vi "MPP.read.vi"(8 "error in (no error)":errorcluster, 11 "VISA Refnum in":refnum<visa-resource-name>) -> (0 "error out":errorcluster, 1 "Impp":dbl, 2 "Vmpp":dbl, 3 "VISA Refnum out":refnum<visa-resource-name>, 4 "Pmpp":dbl)   [LabVIEW 2020, in "main.lvlib"]
uses:
  main.lvlib
  <instrlib>/HH PLA Series/HH PLA Series.lvlib
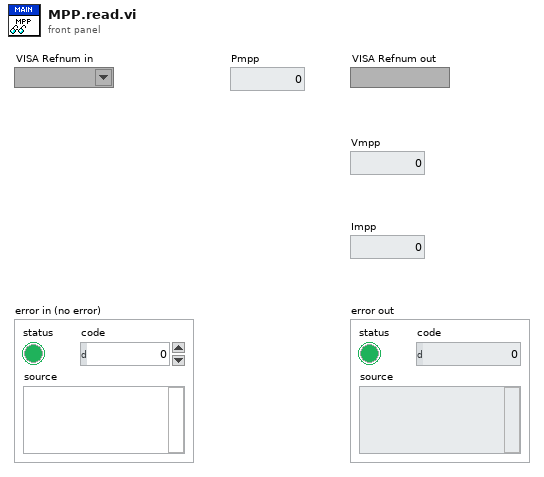
[diagram p1: front panel]
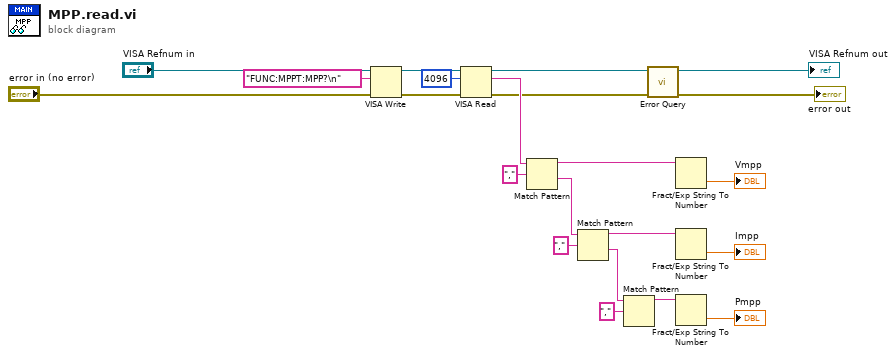
[diagram p0: block diagram]
diagram:
  n1 = VISA Write(VISA resource name="VISA Refnum in", write buffer="FUNC:MPPT:MPP?\n", error in (no error)="error in (no error)") -> (VISA resource name out=w17:refnum<visa-resource-name>, error out=w18:errorcluster)  [unwired: 1 out]
  n2 = VISA Read(VISA resource name=w17, byte count=u32 4096, error in (no error)=w18) -> (VISA resource name out=w4:refnum<visa-resource-name>, read buffer=w20:string, error out=w2:errorcluster)  [unwired: 1 out]
  n3 = Match Pattern(string=w20, regular expression=",") -> (before substring=w6:string, after substring=w9:string)  [unwired: 1 in, 2 out]
  n4 = Match Pattern(string=w9, regular expression=",") -> (before substring=w11:string, after substring=w15:string)  [unwired: 1 in, 2 out]
  n5 = Match Pattern(string=w15, regular expression=",") -> (before substring=w12:string)  [unwired: 1 in, 3 out]
  n6 = call <instrlib>:"Error Query.vi"("error in (no error)"=w2, "VISA resource name"=w4) -> ("error out"=→"error out":errorcluster, "VISA resource name out"=→"VISA Refnum out":refnum<visa-resource-name>)  [unwired: 6 in, 2 out]
  n7 = Fract/Exp String To Number(string=w6) -> (number=→"Vmpp":dbl)  [unwired: 3 in, 1 out]
  n8 = Fract/Exp String To Number(string=w11) -> (number=→"Impp":dbl)  [unwired: 3 in, 1 out]
  n9 = Fract/Exp String To Number(string=w12) -> (number=→"Pmpp":dbl)  [unwired: 3 in, 1 out]
